vi "Parse.vi"(8 "error in (no error)":errorcluster, 10 "Data String":string, 11 "Multi Parser in":refnum<class "Multi Sentence Parser.lvclass">) -> (0 "error out":errorcluster, 2 "Data Values":dbl[](array[numeric]), 3 "Multi Parser out":refnum<class "Multi Sentence Parser.lvclass">)   [LabVIEW 2018, in "Multi Sentence Parser.lvclass"]
doc: "Multi Sentence Parser.lvclass:Parse.vi\n\nThis VI parses multiple strings read from an instrument as input and returns an array of channel values.\n\nInstrument Communication Module Version 1.0\nOctober, 2018 Original Code Consulting David Thomson\n www.originalcode.com"
uses:
  Multi Sentence Parser.lvclass
  Multi Sentence Parser.lvclass/Multi Sentence Parser.ctl
  SubVIs/Parsing VIs/ICM whitespace.ctl
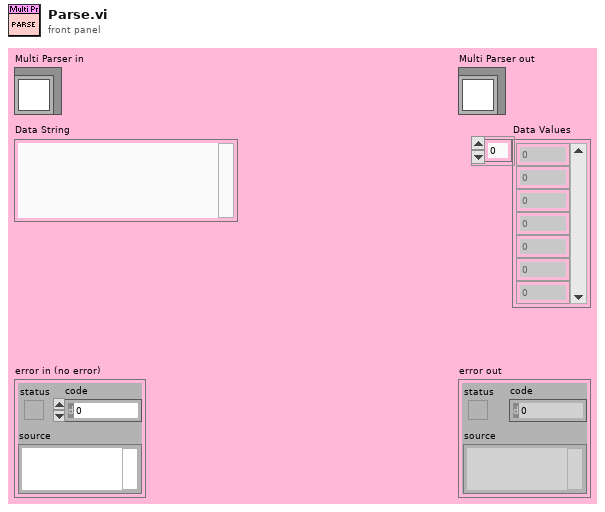
[diagram p1: front panel]
types:
  T1 = cluster{"Sentence ID":string, "Format String":string, "Channels":string[], "Enabled":bool[]}[]
  T2 = cluster{"Sentence ID":string, "Format String":string, "Channels":string[], "Enabled":bool[]}
  T3 = typedef "ICM whitespace.ctl" = u16
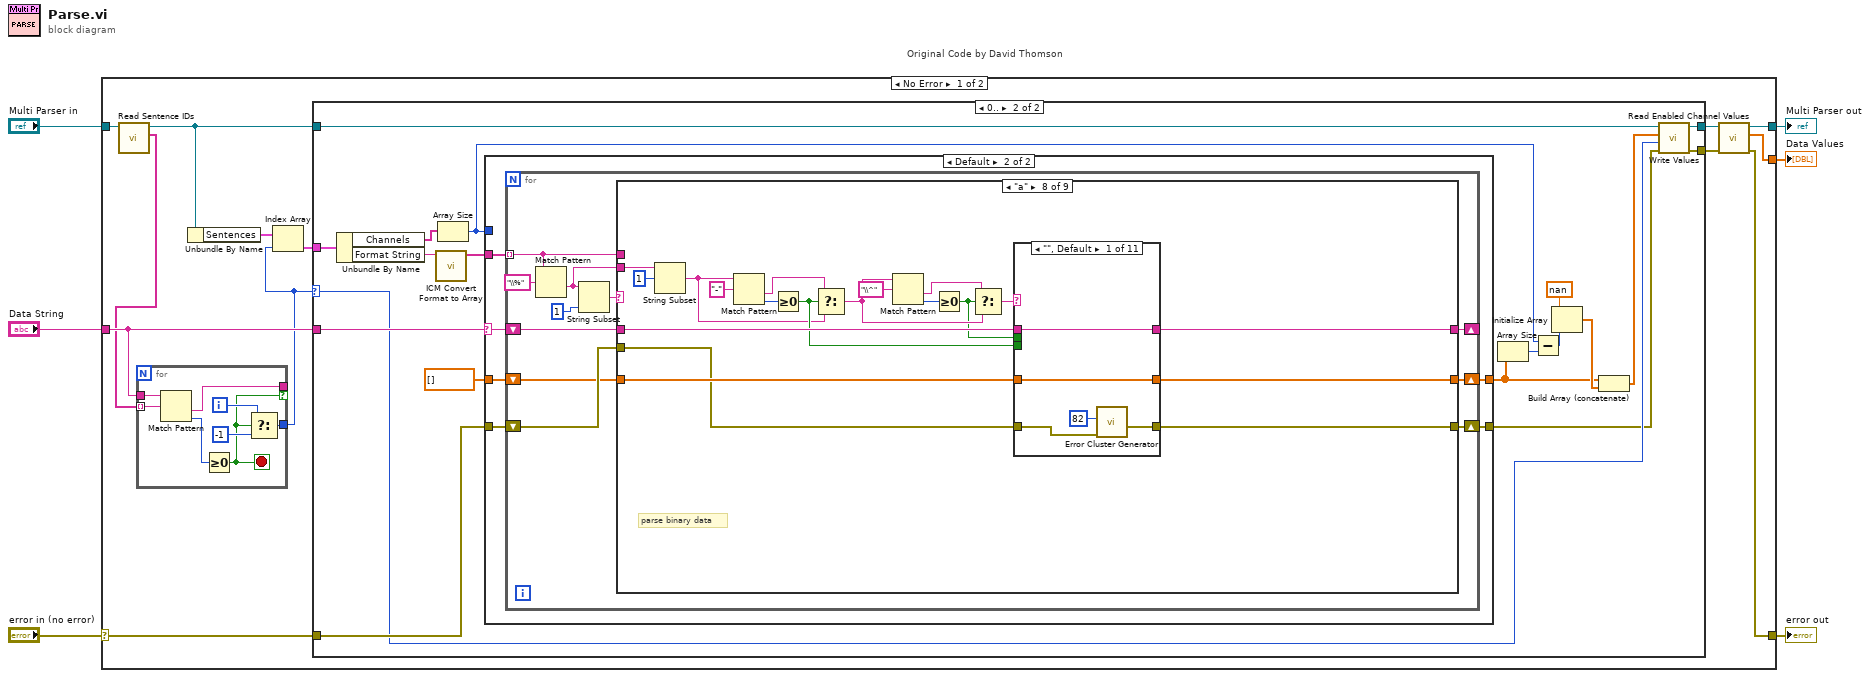
[diagram p0: block diagram]
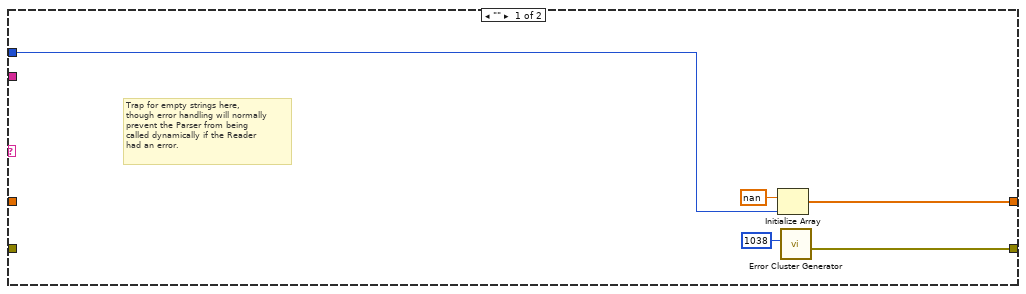
[diagram p3: hidden frame]
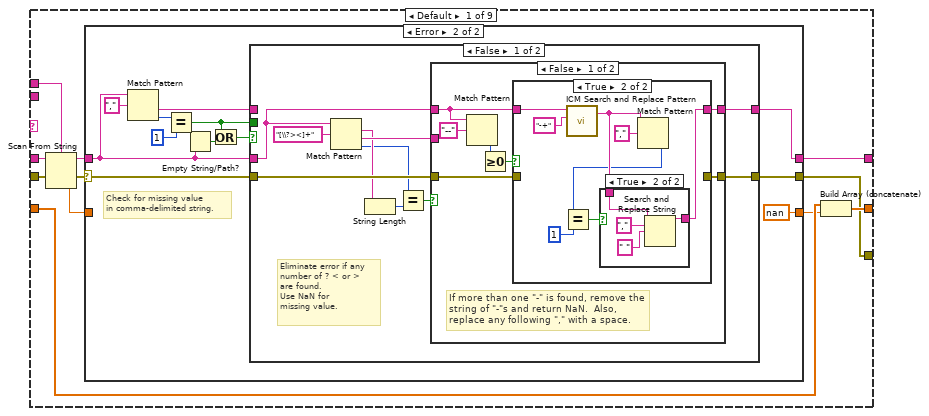
[diagram p4: hidden frame]
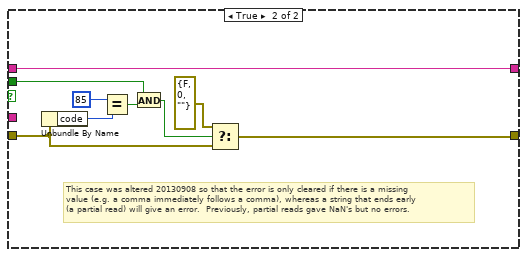
[diagram p9: hidden frame]
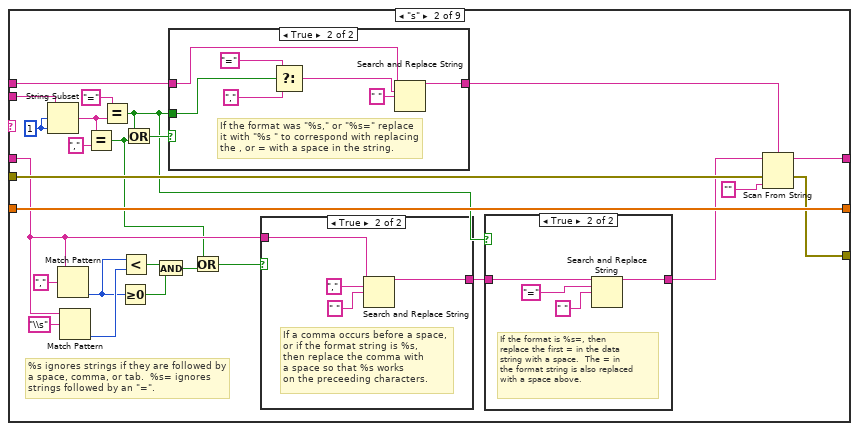
[diagram p10: hidden frame]
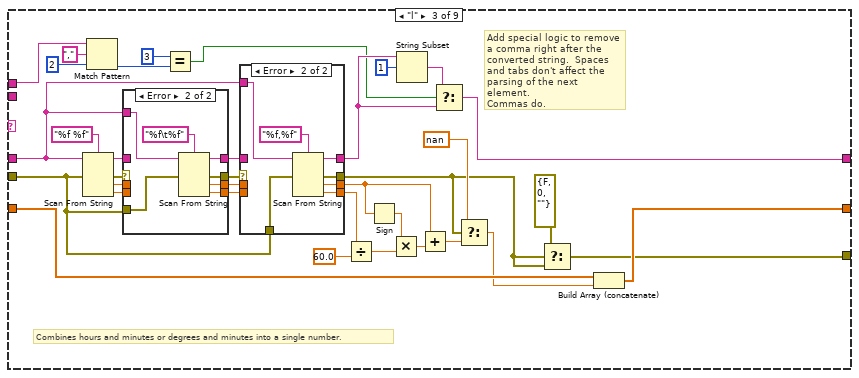
[diagram p14: hidden frame]
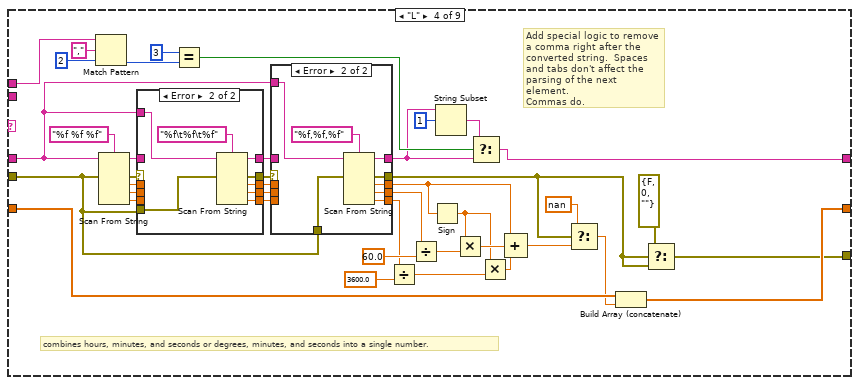
[diagram p17: hidden frame]
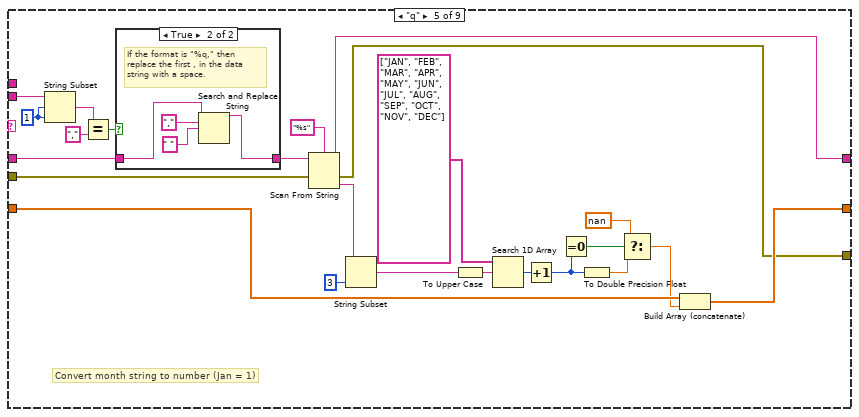
[diagram p20: hidden frame]
diagram:
  n1 = case "Original Code by David Thomson" shown="No Error" "error in (no error)" {
    selector: "error in (no error)" -> [w19 w594]
    tunnel: [w8 w594] -> w5
    tunnel: "Multi Parser in" -> [w18 w593]
    tunnel: "Data String" -> [w16 _]
    tunnel: [w9 _] -> w2
    tunnel: [w11 w593] -> w1
    frame No Error {
      n2 = call-dynamic "Read Sentence IDs.vi"("Multi Parser in"=w18) -> ("Sentence IDs"=w15:string[], "Multi Parser out"=w12:refnum<class "Multi Sentence Parser.lvclass">)  [unwired: 8 in, 1 out]
      n3 = for {
        tunnel: w15 -> [w591] mode=indexing
        tunnel: w16 -> [w592]
        tunnel: [w587] -> w13
        tunnel: [w586] -> _ if=w585
        i -> [w589]
        stop <- w585 stop-if-true
        n4 = Match Pattern(string=w592, regular expression=w591) -> (after substring=w586:string, offset past match=w590:i32)  [unwired: 1 in, 2 out]
        n5 = Greater Or Equal To 0?(x=w590) -> (x >= 0?=w585:bool)
        n6 = Select(t=w589, s=w585, f=-1) -> (s? t:f=w587:i32)
      }
      n7 = Unbundle By Name(w12) -> ("Sentences"=w17:T1)
      n8 = Index Array(array=w17, index=w13) -> (element=w14:T2)
      n9 = case shown="0.." w13 {
        selector: w13 -> [_ w24]
        tunnel: w19 -> [w21 w33]
        tunnel: [w21 w23] -> w7
        tunnel: w16 -> [_ w29]
        tunnel: w14 -> [_ w28]
        tunnel: w12 -> [w20 w26]
        tunnel: [w20 w25] -> w10
        frame ..-1 {
        }
        frame 0.. {
          n10 = Unbundle By Name(w28) -> ("Channels"=w31:string[], "Format String"=w32:string)
          n11 = call "ICM Convert Format to Array.vi"("Format String"=w32) -> ("Format Array"=w34:string[])  [unwired: 10 in]
          n12 = Array Size(array=w31) -> (size(s)=w30:i32)
          n13 = case shown="Default" w29 {
            selector: w29 -> [_ w46]
            tunnel: w33 -> [_ w51]
            tunnel: w34 -> [_ w50]
            tunnel: [w45 w49] -> w22
            tunnel: dbl[] [] ("Values") -> [_ w48]
            tunnel: [w42 w47] -> w35
            tunnel: w30 -> [w41 _]
            frame "" {
              # "Trap for empty strings here,\nthough error handling will normally\nprevent the Parser from being\ncalled dynamically if the Reader\nhad an error."
              n14 = Initialize Array(nan ("y"), w41) -> (w42:dbl[])
              n15 = call "Error Cluster Generator.vi"("code"=1038) -> ("error out"=w45:errorcluster)  [unwired: 5 in, 1 out]
            }
            frame Default {
              n16 = for {
                shift-right: [w55] -> _
                shift-left: w46 -> [w62]
                shift-right: [w56] -> w49
                shift-left: w51 -> [w61]
                tunnel: w50 -> [w53] mode=indexing
                shift-right: [w58] -> w47
                shift-left: w48 -> [w59]
                n17 = Match Pattern(string=w53, regular expression="\\%") -> (after substring=w52:string)  [unwired: 4 out]
                n18 = String Subset(string=w52, length (rest)=1 ("length (rest)")) -> (substring=w57:string)  [unwired: 1 out]
                n19 = case shown="\"a\"" w57 {
                  selector: w57 -> [_ _ _ _ _ w339 _ _ _]
                  tunnel: w62 -> [w73 w145 w192 w256 w300 w329 w434 w455 w546]
                  tunnel: w61 -> [w72 w153 w191 w255 w318 w347 w432 w450 w549]
                  tunnel: w53 -> [w71 w142 w187 w240 _ _ _ _ _]
                  tunnel: [w70 w154 w203 w267 w316 w331 w435 w451 w547] -> w58
                  tunnel: w59 -> [w65 w154 w204 w268 w317 _ w435 w452 w564]
                  tunnel: [w68 w152 w175 w232 w314 w340 w432 w449 w550] -> w56
                  tunnel: [w63 w156 w182 w236 w315 w341 w433 w454 w542] -> w55
                  tunnel: w52 -> [_ w144 _ _ w302 _ w428 w448 w557]
                  frame Default {
                    n20 = Scan From String(format string=w71, input string=w73, error in=w72) -> (remaining string=w67:string, error out=w69:errorcluster, output 1=w66:dbl)  [unwired: 1 in, 2 out]
                    n21 = case shown="Error" w69 {
                      selector: w69 -> [w76 w84]
                      tunnel: [w76 w78] -> w68
                      tunnel: [w75 w79] -> w63
                      tunnel: w67 -> [w75 w80]
                      tunnel: w66 -> [w74 _]
                      tunnel: [w74 nan ("y")] -> w64
                      frame No Error {
                        # "this case uses LabVIEW's built in parsing codes"
                      }
                      frame Error {
                        # "Check for missing value\nin comma-delimited string."
                        n22 = Match Pattern(string=w80, regular expression=",") -> (after substring=w85:string, offset past match=w87:i32)  [unwired: 3 out]
                        n23 = Equal?(x=w87, y=1) -> (x = y?=w77:bool)
                        n24 = Empty String/Path?(string/path=w80) -> (empty?=w81:bool)
                        n25 = Or(x=w77, y=w81) -> (x .or. y?=w82:bool)
                        n26 = case shown="False" w82 {
                          tunnel: [w94 w130] -> w79
                          tunnel: w85 -> [_ w130]
                          tunnel: w80 -> [w96 _]
                          tunnel: [w93 w129] -> w78
                          tunnel: w84 -> [w95 w128]
                          tunnel: w77 -> [_ w123]
                          frame False {
                            # "Eliminate error if any\nnumber of ? < or >\nare found.\nUse NaN for\nmissing value."
                            n27 = Match Pattern(string=w96, regular expression="[\\?><]+") -> (match substring=w91:string, after substring=w92:string, offset past match=w89:i32)  [unwired: 2 out]
                            n28 = String Length(string=w91) -> (length=w90:i32)
                            n29 = Equal?(x=w89, y=w90) -> (x = y?=w97:bool)
                            n30 = case shown="False" w97 {
                              tunnel: [w100 w121] -> w94
                              tunnel: w96 -> [w99 _]
                              tunnel: [w101 _] -> w93
                              tunnel: w95 -> [w102 _]
                              tunnel: w92 -> [_ w121]
                              frame False {
                                # "If more than one \"-\" is found, remove the\nstring of \"-\"s and return NaN.  Also,\nreplace any following \",\" with a space."
                                n31 = Match Pattern(string=w99, regular expression="--") -> (offset past match=w104:i32)  [unwired: 4 out]
                                n32 = Greater Or Equal To 0?(x=w104) -> (x >= 0?=w103:bool)
                                n33 = case shown="True" w103 {
                                tunnel: [w107 _] -> w101
                                tunnel: w102 -> [w107 _]
                                tunnel: [w106 w113] -> w100
                                tunnel: w99 -> [w106 w115]
                                frame False {
                                }
                                frame True {
                                n34 = call "ICM Search and Replace Pattern.vi"("string"=w115, "regular expression (\"\")"="-+" ("regular expression (\"\")")) -> ("result string"=w111:string)  [unwired: 1 in, 3 out]
                                n35 = Match Pattern(string=w111, regular expression=",") -> (offset past match=w109:i32)  [unwired: 4 out]
                                n36 = Equal?(x=w109, y=1) -> (x = y?=w108:bool)
                                n37 = case shown="True" w108 {
                                tunnel: w111 -> [w116 w118]
                                tunnel: [w116 w117] -> w113
                                frame False {
                                }
                                frame True {
                                n38 = Search and Replace String(input string=w118, search string=",", replace string=" " ("replace string (\"\")")) -> (result string=w117:string)  [unwired: 1 in, 7 out]
                                }
                                }
                                }
                                }
                              }
                              frame True {
                              }
                            }
                          }
                          frame True {
                            # "This case was altered 20130908 so that the error is only cleared if there is a missing\nvalue (e.g. a comma immediately follows a comma), whereas a string that ends early\n(a partial read) will give an error.  Previously, partial reads gave NaN's but no errors."
                            n39 = Unbundle By Name(w128) -> ("code"=w127:i32)
                            n40 = Equal?(x=85, y=w127) -> (x = y?=w124:bool)
                            n41 = And(x=w123, y=w124) -> (x .and. y?=w122:bool)
                            n42 = Select(t=errorcluster {"status"=FALSE, "code"=0, "source"=""}, s=w122, f=w128) -> (s? t:f=w129:errorcluster)
                          }
                        }
                      }
                    }
                    n43 = Build Array (concatenate)(w65, w64) -> (w70:dbl[])
                  }
                  frame "s" {
                    w140 = 1 ("length (rest)")
                    # "%s ignores strings if they are followed by\na space, comma, or tab.  %s= ignores\nstrings followed by an \"=\"."
                    n44 = String Subset(string=w144, offset (0)=w140, length (rest)=w140) -> (substring=w138:string)
                    n45 = Match Pattern(string=w145, regular expression=",") -> (offset past match=w147:i32)  [unwired: 4 out]
                    n46 = Match Pattern(string=w145, regular expression="\\s") -> (offset past match=w149:i32)  [unwired: 4 out]
                    n47 = Equal?(x=w138, y=",") -> (x = y?=w132:bool)
                    n48 = Equal?(x="=" ("y"), y=w138) -> (x = y?=w134:bool)
                    n49 = Greater Or Equal To 0?(x=w147) -> (x >= 0?=w146:bool)
                    n50 = Less?(x=w147, y=w149) -> (x < y?=w148:bool)
                    n51 = Or(x=w134, y=w132) -> (x .or. y?=w139:bool)
                    n52 = And(x=w148, y=w146) -> (x .and. y?=w133:bool)
                    n53 = case shown="True" w139 {
                      tunnel: [w162 w167] -> w141
                      tunnel: w142 -> [w162 w168]
                      tunnel: w134 -> [_ w163]
                      frame False {
                      }
                      frame True {
                        # "If the format was \"%s,\" or \"%s=\" replace\nit with \"%s \" to correspond with replacing\nthe , or = with a space in the string."
                        n54 = Select(t="=" ("y"), s=w163, f="," ("search string")) -> (s? t:f=w164:string)
                        n55 = Search and Replace String(input string=w168, search string=w164, replace string=" " ("replace string (\"\")")) -> (result string=w167:string)  [unwired: 1 in, 7 out]
                      }
                    }
                    n56 = Or(x=w132, y=w133) -> (x .or. y?=w131:bool)
                    n57 = case shown="True" w131 {
                      tunnel: [w170 w172] -> w136
                      tunnel: w145 -> [w170 w171]
                      frame False {
                      }
                      frame True {
                        # "If a comma occurs before a space, \nor if the format string is %s,\nthen replace the comma with\na space so that %s works\non the preceeding characters."
                        n58 = Search and Replace String(input string=w171, search string=",", replace string=" " ("replace string (\"\")")) -> (result string=w172:string)  [unwired: 1 in, 7 out]
                      }
                    }
                    n59 = case shown="True" w134 {
                      tunnel: w136 -> [w157 w159]
                      tunnel: [w157 w158] -> w135
                      frame False {
                      }
                      frame True {
                        # "If the format is %s=, then\nreplace the first = in the data\nstring with a space.  The = in\nthe format string is also replaced\nwith a space above."
                        n60 = Search and Replace String(input string=w159, search string="=", replace string=" " ("replace string (\"\")")) -> (result string=w158:string)  [unwired: 1 in, 7 out]
                      }
                    }
                    n61 = Scan From String(format string=w141, input string=w135, error in=w153, default 1="") -> (remaining string=w156:string, error out=w152:errorcluster)  [unwired: 1 in, 2 out]
                  }
                  frame "l" {
                    # "Combines hours and minutes or degrees and minutes into a single number."
                    # "Add special logic to remove\na comma right after the\nconverted string.  Spaces\nand tabs don't affect the\nparsing of the next element.\nCommas do."
                    n62 = Scan From String(format string="%f %f", input string=w192, error in=w191) -> (remaining string=w199:string, error out=w202:errorcluster, output 1=w201:dbl, output 2=w200:dbl)  [unwired: 1 in, 3 out]
                    n63 = Match Pattern(string=w187, regular expression=",", offset (0)=2) -> (offset past match=w180:i32)  [unwired: 3 out]
                    n64 = case shown="Error" w202 {
                      selector: w202 -> [w224 _]
                      tunnel: [w224 w225] -> w198
                      tunnel: [w223 w230] -> w197
                      tunnel: w201 -> [w223 _]
                      tunnel: [w222 w229] -> w196
                      tunnel: w200 -> [w222 _]
                      tunnel: w199 -> [w221 _]
                      tunnel: [w221 w228] -> w193
                      tunnel: w192 -> [_ w227]
                      tunnel: w191 -> [_ w226]
                      frame No Error {
                      }
                      frame Error {
                        n65 = Scan From String(format string="%f\t%f", input string=w227, error in=w226) -> (remaining string=w228:string, error out=w225:errorcluster, output 1=w230:dbl, output 2=w229:dbl)  [unwired: 1 in, 3 out]
                      }
                    }
                    n66 = Equal?(x=3, y=w180) -> (x = y?=w179:bool)
                    n67 = case shown="Error" w198 {
                      selector: w198 -> [w213 _]
                      tunnel: [w213 w217] -> w176
                      tunnel: [w212 w219] -> w195
                      tunnel: w197 -> [w212 _]
                      tunnel: [w211 w218] -> w194
                      tunnel: w196 -> [w211 _]
                      tunnel: w193 -> [w210 _]
                      tunnel: [w210 w216] -> w181
                      tunnel: w192 -> [_ w215]
                      tunnel: w191 -> [_ w214]
                      frame No Error {
                      }
                      frame Error {
                        n68 = Scan From String(format string="%f,%f", input string=w215, error in=w214) -> (remaining string=w216:string, error out=w217:errorcluster, output 1=w219:dbl, output 2=w218:dbl)  [unwired: 1 in, 3 out]
                      }
                    }
                    n69 = Divide(x=w194, y=60.0) -> (x/y=w207:dbl)
                    n70 = Sign(1:w195) -> (0:w206:dbl)
                    n71 = Multiply(x=w206, y=w207) -> (x*y=w205:dbl)
                    n72 = String Subset(string=w181, offset (0)=1) -> (substring=w183:string)  [unwired: 1 out]
                    n73 = Add(x=w195, y=w205) -> (x+y=w190:dbl)
                    n74 = Select(t=w183, s=w179, f=w181) -> (s? t:f=w182:string)
                    n75 = Select(t=nan ("y"), s=w176, f=w190) -> (s? t:f=w189:dbl)
                    n76 = Select(t=errorcluster {"status"=FALSE, "code"=0, "source"=""}, s=w176, f=w176) -> (s? t:f=w175:errorcluster)
                    n77 = Build Array (concatenate)(w204, w189) -> (w203:dbl[])
                  }
                  frame "L" {
                    # "combines hours, minutes, and seconds or degrees, minutes, and seconds into a single number."
                    # "Add special logic to remove\na comma right after the\nconverted string.  Spaces\nand tabs don't affect the\nparsing of the next element.\nCommas do."
                    n78 = Match Pattern(string=w240, regular expression=",", offset (0)=2) -> (offset past match=w242:i32)  [unwired: 3 out]
                    n79 = Scan From String(format string="%f %f %f", input string=w256, error in=w255) -> (remaining string=w263:string, error out=w266:errorcluster, output 1=w265:dbl, output 2=w264:dbl, output 3=w251:dbl)  [unwired: 1 in, 4 out]
                    n80 = case shown="Error" w266 {
                      selector: w266 -> [w290 _]
                      tunnel: [w290 w292] -> w262
                      tunnel: [w289 w297] -> w261
                      tunnel: w265 -> [w289 _]
                      tunnel: [w288 w296] -> w260
                      tunnel: w264 -> [w288 _]
                      tunnel: w263 -> [w287 _]
                      tunnel: [w287 w295] -> w257
                      tunnel: w256 -> [_ w294]
                      tunnel: w255 -> [_ w293]
                      tunnel: w251 -> [w286 _]
                      tunnel: [w286 w291] -> w250
                      frame No Error {
                      }
                      frame Error {
                        n81 = Scan From String(format string="%f\t%f\t%f", input string=w294, error in=w293) -> (remaining string=w295:string, error out=w292:errorcluster, output 1=w297:dbl, output 2=w296:dbl, output 3=w291:dbl)  [unwired: 1 in, 4 out]
                      }
                    }
                    n82 = Equal?(x=3, y=w242) -> (x = y?=w237:bool)
                    n83 = case shown="Error" w262 {
                      selector: w262 -> [w277 _]
                      tunnel: [w277 w282] -> w233
                      tunnel: [w276 w284] -> w259
                      tunnel: w261 -> [w276 _]
                      tunnel: [w275 w283] -> w258
                      tunnel: w260 -> [w275 _]
                      tunnel: w257 -> [w274 _]
                      tunnel: [w274 w281] -> w235
                      tunnel: w256 -> [_ w280]
                      tunnel: w255 -> [_ w279]
                      tunnel: [w273 w278] -> w247
                      tunnel: w250 -> [w273 _]
                      frame No Error {
                      }
                      frame Error {
                        n84 = Scan From String(format string="%f,%f,%f", input string=w280, error in=w279) -> (remaining string=w281:string, error out=w282:errorcluster, output 1=w284:dbl, output 2=w283:dbl, output 3=w278:dbl)  [unwired: 1 in, 4 out]
                      }
                    }
                    n85 = Divide(x=w247, y=3600.0) -> (x/y=w249:dbl)
                    n86 = Divide(x=w258, y=60.0) -> (x/y=w270:dbl)
                    n87 = Sign(1:w259) -> (0:w246:dbl)
                    n88 = String Subset(string=w235, offset (0)=1) -> (substring=w238:string)  [unwired: 1 out]
                    n89 = Multiply(x=w246, y=w270) -> (x*y=w269:dbl)
                    n90 = Select(t=w238, s=w237, f=w235) -> (s? t:f=w236:string)
                    n91 = Multiply(x=w246, y=w249) -> (x*y=w245:dbl)
                    n92 = Compound Arithmetic op=ADD(w259, w269, w245) -> (w254:dbl)
                    n93 = Select(t=nan ("y"), s=w233, f=w254) -> (s? t:f=w253:dbl)
                    n94 = Build Array (concatenate)(w268, w253) -> (w267:dbl[])
                    n95 = Select(t=errorcluster {"status"=FALSE, "code"=0, "source"=""}, s=w233, f=w233) -> (s? t:f=w232:errorcluster)
                  }
                  frame "q" {
                    w304 = 1 ("length (rest)")
                    # "Convert month string to number (Jan = 1)"
                    n96 = String Subset(string=w302, offset (0)=w304, length (rest)=w304) -> (substring=w303:string)
                    n97 = Equal?(x=w303, y=",") -> (x = y?=w301:bool)
                    n98 = case shown="True" w301 {
                      tunnel: w300 -> [w323 w325]
                      tunnel: [w323 w324] -> w299
                      frame False {
                      }
                      frame True {
                        # "If the format is \"%q,\" then\nreplace the first , in the data\nstring with a space."
                        n99 = Search and Replace String(input string=w325, search string=",", replace string=" " ("replace string (\"\")")) -> (result string=w324:string)  [unwired: 1 in, 7 out]
                      }
                    }
                    n100 = Scan From String(format string="%s", input string=w299, error in=w318) -> (remaining string=w315:string, error out=w314:errorcluster, output 1=w313:string)  [unwired: 1 in, 2 out]
                    n101 = String Subset(string=w313, length (rest)=3 ("length (rest)")) -> (substring=w311:string)  [unwired: 1 out]
                    n102 = To Upper Case(1:w311) -> (0:w320:string)
                    n103 = Search 1D Array(1D array=string[] ["JAN", "FEB", "MAR", "APR", "MAY", "JUN", "JUL", "AUG", "SEP", "OCT", "NOV", "DEC"], element=w320) -> (index of element=w322:i32)  [unwired: 1 out]
                    n104 = Increment(x=w322) -> (x+1=w310:i32)
                    n105 = Equal To 0?(x=w310) -> (x = 0?=w309:bool)
                    n106 = To Double Precision Float(number=w310) -> (double precision float=w308:dbl)
                    n107 = Select(t=nan ("y"), s=w309, f=w308) -> (s? t:f=w307:dbl)
                    n108 = Build Array (concatenate)(w317, w307) -> (w316:dbl[])
                  }
                  frame "I", "i" {
                    w328 = T3 1 items=["both", "start of string", "end of string"] ("location (both)")
                    # "decodes ISO 8601 time strings\n\"I\" includes a time stamp before\nthe other channels"
                    n109 = call "ICM Trim Whitespace.vi"("string"=w329, "location (both)"=w328) -> ("trimmed string"=w330:string)
                    n110 = Match Pattern(string=w330, regular expression="[T\\s]") -> (before substring=w348:string, after substring=w343:string)  [unwired: 3 out]
                    n111 = Match Pattern(string=w343, regular expression="[\\s\\t,]") -> (before substring=w342:string, after substring=w341:string)  [unwired: 3 out]
                    n112 = Match Pattern(string=w348, regular expression="-") -> (offset past match=w349:i32)  [unwired: 4 out]
                    n113 = case "Decode Date" shown="5" w349 {
                      tunnel: w348 -> [w407 w420]
                      tunnel: [w404 w417] -> w333
                      tunnel: [w399 w416] -> w332
                      tunnel: [w405 w418] -> w334
                      tunnel: w347 -> [w398 w414]
                      tunnel: [w395 w413] -> w335
                      frame 0, Default {
                        w401 = 0.0 ("default value 1")
                        w400 = "%d" ("format string")
                        n114 = String Subset(string=w407, length (rest)=4 ("length (rest)")) -> (substring=w406:string)  [unwired: 1 out]
                        n115 = String Subset(string=w407, offset (0)=4, length (rest)=2 ("length (rest)")) -> (substring=w403:string)
                        n116 = String Subset(string=w407, offset (0)=6, length (rest)=2 ("length (rest)")) -> (substring=w402:string)
                        n117 = Scan From String(format string=w400, input string=w402, error in=w398, default 1=w401) -> (error out=w397:errorcluster, output 1=w399:dbl)  [unwired: 1 in, 2 out]
                        n118 = Scan From String(format string=w400, input string=w403, error in=w397, default 1=w401) -> (error out=w396:errorcluster, output 1=w404:dbl)  [unwired: 1 in, 2 out]
                        n119 = Scan From String(format string=w400, input string=w406, error in=w396, default 1=w401) -> (error out=w395:errorcluster, output 1=w405:dbl)  [unwired: 1 in, 2 out]
                      }
                      frame 5 {
                        w415 = 0.0 ("default value 1")
                        n120 = Scan From String(format string="%d-%d-%d", input string=w420, error in=w414, default 1=w415, default 2=w415, default 3=w415) -> (error out=w413:errorcluster, output 1=w418:dbl, output 2=w417:dbl, output 3=w416:dbl)  [unwired: 1 in, 2 out]
                      }
                    }
                    n121 = Match Pattern(string=w342, regular expression=":") -> (offset past match=w345:i32)  [unwired: 4 out]
                    n122 = case "Decode Time" shown="3" w345 {
                      tunnel: w342 -> [w381 w394]
                      tunnel: [w379 w391] -> w337
                      tunnel: [w374 w390] -> w336
                      tunnel: [w368 w392] -> w338
                      tunnel: w335 -> [w373 w388]
                      tunnel: [w370 w387] -> w340
                      frame 0, Default {
                        w376 = 0.0 ("default value 1")
                        w375 = "%d" ("format string")
                        n123 = String Subset(string=w381, length (rest)=2 ("length (rest)")) -> (substring=w380:string)  [unwired: 1 out]
                        n124 = String Subset(string=w381, offset (0)=2, length (rest)=2 ("length (rest)")) -> (substring=w378:string)
                        n125 = String Subset(string=w381, offset (0)=4, length (rest)=2 ("length (rest)")) -> (substring=w377:string)
                        n126 = Scan From String(format string="%f", input string=w377, error in=w373, default 1=w376) -> (error out=w372:errorcluster, output 1=w374:dbl)  [unwired: 1 in, 2 out]
                        n127 = Scan From String(format string=w375, input string=w378, error in=w372, default 1=w376) -> (error out=w371:errorcluster, output 1=w379:dbl)  [unwired: 1 in, 2 out]
                        n128 = Scan From String(format string=w375, input string=w380, error in=w371, default 1=w376) -> (error out=w370:errorcluster, output 1=w368:dbl)  [unwired: 1 in, 2 out]
                      }
                      frame 3 {
                        w389 = 0.0 ("default value 1")
                        n129 = Scan From String(format string="%d:%d:%f", input string=w394, error in=w388, default 1=w389, default 2=w389, default 3=w389) -> (error out=w387:errorcluster, output 1=w392:dbl, output 2=w391:dbl, output 3=w390:dbl)  [unwired: 1 in, 2 out]
                      }
                    }
                    n130 = case shown="\"I\"" w339 {
                      tunnel: w338 -> [w355 w367]
                      tunnel: w337 -> [w354 w362]
                      tunnel: w336 -> [w353 w363]
                      tunnel: w334 -> [w358 w359]
                      tunnel: w333 -> [w357 w360]
                      tunnel: w332 -> [w356 w361]
                      tunnel: [w352 w366] -> w331
                      frame "i", Default {
                        n131 = Build Array(w358, w357, w356, w355, w354, w353) -> (w352:dbl[])
                      }
                      frame "I" {
                        n132 = call "ICM Calculate Time Stamps.vi"("Second"=w363, "Year"=w359, "Minute"=w362, "Hour"=w362, "Day"=w361, "Month"=w360) -> ("Seconds Since Midnight"=w365:dbl, "TimeStamp"=w364:dbl)  [unwired: 4 in]
                        n133 = Build Array(w364, w365, w359, w360, w361, w367, w362, w363) -> (w366:dbl[])
                      }
                    }
                  }
                  frame "z" {
                    w425 = "," ("regular expression")
                    # "special case for %z with no \"n\" following it - skip one character"
                    # "%zn ignores n characters"
                    n134 = Match Pattern(string=w428, regular expression=w425) -> (before substring=w427:string, match substring=w426:string)  [unwired: 3 out]
                    n135 = Equal?(x=w426, y=w425) -> (x = y?=w423:bool)
                    n136 = String Length(string=w427) -> (length=w430:i32)
                    n137 = Greater?(x=w430, y=1) -> (0:w431:bool)
                    n138 = case shown="True" w431 {
                      tunnel: w427 -> [_ w439]
                      tunnel: [1 w437] -> w422
                      frame False {
                      }
                      frame True {
                        n139 = Scan From String(format string="z%d", input string=w439) -> (output 1=w437:i32)  [unwired: 2 in, 4 out]
                      }
                    }
                    n140 = Increment(x=w422) -> (x+1=w421:i32)
                    n141 = Select(t=w421, s=w423, f=w422) -> (s? t:f=w424:i32)
                    n142 = String Subset(string=w434, offset (0)=w424) -> (substring=w433:string)  [unwired: 1 out]
                  }
                  frame "a" {
                    # "parse binary data"
                    n143 = String Subset(string=w448, offset (0)=1) -> (substring=w447:string)  [unwired: 1 out]
                    n144 = Match Pattern(string=w447, regular expression="-") -> (after substring=w456:string, offset past match=w457:i32)  [unwired: 3 out]
                    n145 = Greater Or Equal To 0?(x=w457) -> (x >= 0?=w453:bool)
                    n146 = Select(t=w456, s=w453, f=w447) -> (s? t:f=w441:string)
                    n147 = Match Pattern(string=w441, regular expression="\\^") -> (after substring=w444:string, offset past match=w442:i32)  [unwired: 3 out]
                    n148 = Greater Or Equal To 0?(x=w442) -> (x >= 0?=w440:bool)
                    n149 = Select(t=w444, s=w440, f=w441) -> (s? t:f=w443:string)
                    n150 = case shown="\"\", Default" w443 {
                      tunnel: w455 -> [w463 w469 w478 w486 w494 w500 w509 w517 w525 w533 w541]
                      tunnel: [w463 w468 w477 w485 w493 w499 w508 w516 w524 w532 w540] -> w454
                      tunnel: w453 -> [_ _ w472 w484 w492 _ w503 w515 w523 w531 w539]
                      tunnel: w452 -> [w462 w467 w476 w483 w491 w498 w507 w514 w522 w530 w538]
                      tunnel: [w462 w465 w474 w481 w489 w496 w505 w512 w520 w528 w536] -> w451
                      tunnel: [w461 w464 w473 w480 w488 w495 w504 w511 w519 w527 w535] -> w449
                      tunnel: w450 -> [w460 w464 w473 w480 w488 w495 w504 w511 w519 w527 w535]
                      tunnel: w440 -> [_ _ w471 w479 w487 _ w502 w510 w518 w526 w534]
                      frame "", Default {
                        n151 = call "Error Cluster Generator.vi"("error in"=w460, "code"=82) -> ("error out"=w461:errorcluster)  [unwired: 4 in, 1 out]
                      }
                      frame "U8" {
                        n152 = call "ICM aU8.vi"("String In"=w469) -> ("Value"=w466:dbl, "String Out"=w468:string)  [unwired: 1 in, 8 out]
                        n153 = Build Array (concatenate)(w467, w466) -> (w465:dbl[])
                      }
                      frame "U16" {
                        n154 = Or(x=w471, y=w472) -> (x .or. y?=w470:bool)
                        n155 = call "ICM aU16.vi"("Reverse Bytes"=w470, "String In"=w478) -> ("Value"=w475:dbl, "String Out"=w477:string)  [unwired: 8 out]
                        n156 = Build Array (concatenate)(w476, w475) -> (w474:dbl[])
                      }
                      frame "U32" {
                        n157 = call "ICM aU32.vi"("Reverse Bytes"=w484, "Swap Bytes"=w479, "String In"=w486) -> ("Value"=w482:dbl, "String Out"=w485:string)  [unwired: 1 in, 6 out]
                        n158 = Build Array (concatenate)(w483, w482) -> (w481:dbl[])
                      }
                      frame "U64" {
                        n159 = call "ICM aU64.vi"("Reverse Bytes"=w492, "Swap Bytes"=w487, "String In"=w494) -> ("Value"=w490:dbl, "String Out"=w493:string)  [unwired: 7 out]
                        n160 = Build Array (concatenate)(w491, w490) -> (w489:dbl[])
                      }
                      frame "I8" {
                        n161 = call "ICM aI8.vi"("String In"=w500) -> ("Value"=w497:dbl, "String Out"=w499:string)  [unwired: 1 in, 8 out]
                        n162 = Build Array (concatenate)(w498, w497) -> (w496:dbl[])
                      }
                      frame "I16" {
                        n163 = Or(x=w502, y=w503) -> (x .or. y?=w501:bool)
                        n164 = call "ICM aI16.vi"("Swap Bytes"=w501, "String In"=w509) -> ("Value"=w506:dbl, "String Out"=w508:string)  [unwired: 8 out]
                        n165 = Build Array (concatenate)(w507, w506) -> (w505:dbl[])
                      }
                      frame "I32" {
                        n166 = call "ICM aI32.vi"("Reverse Bytes"=w515, "Swap Bytes"=w510, "String In"=w517) -> ("Value"=w513:dbl, "String Out"=w516:string)  [unwired: 7 out]
                        n167 = Build Array (concatenate)(w514, w513) -> (w512:dbl[])
                      }
                      frame "I64" {
                        n168 = call "ICM aI64.vi"("Reverse Bytes"=w523, "Swap Bytes"=w518, "String In"=w525) -> ("Value"=w521:dbl, "String Out"=w524:string)  [unwired: 7 out]
                        n169 = Build Array (concatenate)(w522, w521) -> (w520:dbl[])
                      }
                      frame "SGL" {
                        n170 = call "ICM aSGL.vi"("Reverse Bytes"=w531, "Swap Bytes"=w526, "String In"=w533) -> ("Value"=w529:dbl, "String Out"=w532:string)  [unwired: 7 out]
                        n171 = Build Array (concatenate)(w530, w529) -> (w528:dbl[])
                      }
                      frame "DBL" {
                        n172 = call "ICM aDBL.vi"("Reverse Bytes"=w539, "Swap Bytes"=w534, "String In"=w541) -> ("Value"=w537:dbl, "String Out"=w540:string)  [unwired: 7 out]
                        n173 = Build Array (concatenate)(w538, w537) -> (w536:dbl[])
                      }
                    }
                  }
                  frame "c" {
                    # "scale the previous channel by a polynomial"
                    n174 = Delete From Array(array=w564) -> (deleted portion=w544:dbl, array with subset deleted=w548:dbl[])  [unwired: 2 in]
                    n175 = Match Pattern(string=w557, regular expression="\\[", offset (0)=1) -> (after substring=w563:string, offset past match=w555:i32)  [unwired: 2 out]
                    n176 = Match Pattern(string=w563, regular expression="\\]") -> (before substring=w561:string, offset past match=w553:i32)  [unwired: 3 out]
                    n177 = Spreadsheet String To Array(delimiter (Tab)=",", format string="%f", spreadsheet string=w561, array type (2D Dbl)=dbl[] []) -> (array=w545:dbl[])
                    n178 = Less Than 0?(x=w555) -> (x < 0?=w554:bool)
                    n179 = Less Than 0?(x=w553) -> (x < 0?=w552:bool)
                    n180 = Or(x=w554, y=w552) -> (x .or. y?=w551:bool)
                    n181 = case shown="False" w551 {
                      tunnel: [w572 w583] -> w550
                      tunnel: w549 -> [w572 w582]
                      tunnel: [w571 w581] -> w547
                      tunnel: w548 -> [w570 w581]
                      tunnel: w546 -> [w569 w580]
                      tunnel: [w569 w580] -> w542
                      tunnel: w545 -> [w568 _]
                      tunnel: w544 -> [w567 _]
                      frame False {
                        n182 = for {
                          tunnel: w568 -> [w579] mode=indexing
                          tunnel: w567 -> [w575]
                          shift-right: [w578] -> w565
                          shift-left: 0.0 ("Numeric") -> [w576]
                          i -> [w574]
                          n183 = Power Of X(1:w575, 2:w574) -> (0:w573:dbl)
                          n184 = Multiply(x=w579, y=w573) -> (x*y=w577:dbl)
                          n185 = Add(x=w577, y=w576) -> (x+y=w578:dbl)
                        }
                        n186 = Build Array (concatenate)(w570, w565) -> (w571:dbl[])
                      }
                      frame True {
                        n187 = call "Error Cluster Generator.vi"("error in"=w582, "code"=82) -> ("error out"=w583:errorcluster)  [unwired: 2 in, 3 out]
                      }
                    }
                  }
                }
              }
            }
          }
          n188 = Array Size(array=w35) -> (size(s)=w38:i32)
          n189 = Subtract(x=w30, y=w38) -> (x-y=w37:i32)
          n190 = Initialize Array(nan ("y"), w37) -> (w36:dbl[])
          n191 = Build Array (concatenate)(w35, w36) -> (w27:dbl[])
          n192 = call-dynamic "Write Values.vi"("error in (no error)"=w22, "Sentence Index"=w24, "Values"=w27, "Multi Parser in"=w26) -> ("error out"=w23:errorcluster, "Multi Parser out"=w25:refnum<class "Multi Sentence Parser.lvclass">)  [unwired: 6 in]
        }
      }
      n193 = call-dynamic "Read Enabled Channel Values.vi"("error in (no error)"=w7, "Multi Parser in"=w10) -> ("error out"=w8:errorcluster, "Enabled Values"=w9:dbl[], "Multi Parser out"=w11:refnum<class "Multi Sentence Parser.lvclass">)  [unwired: 7 in]
    }
    frame Error {
    }
  }
  "error out" <- w5
  "Multi Parser out" <- w1
  "Data Values" <- w2
